vi "New Digital Edge Trigger.vi"(7 "Slope":T1, 8 "error in (no error)":errorcluster) -> (0 "error out":errorcluster, 3 "Digital Edge Trigger out":refnum<class "Digital Edge Trigger.lvclass">)   [LabVIEW 2015, in "Waveform Data Logger Engine.lvlib" / "Digital Edge Trigger.lvclass"]
uses:
  Digital Edge Trigger.lvclass
  Digital Slope Type.ctl
  Digital Edge Trigger.lvclass/Digital Edge Trigger.ctl
  Trigger/Trigger Type.ctl
  Trigger/Trigger.lvclass/Trigger.ctl
  Trigger/Write Trigger Type.vi
  Trigger/Trigger.lvclass
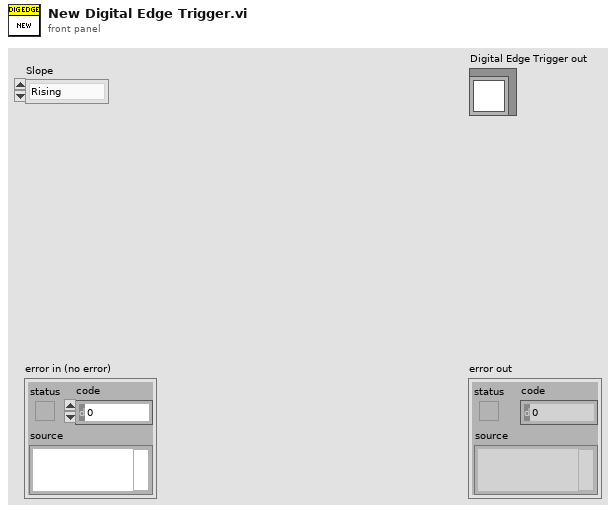
[diagram p1: front panel]
types:
  T1 = typedef "Waveform Data Logger Engine.lvlib/Digital Edge Trigger.lvclass/Digital Slope Type.ctl" = enum16{"Rising", "Falling"}
  T2 = typedef "Waveform Data Logger Engine.lvlib/Trigger.lvclass/Trigger Type.ctl" = enum16{"Default", "Digital Edge", "Analog Edge", "In Range", "Value Change", "Boolean Evaluation"}
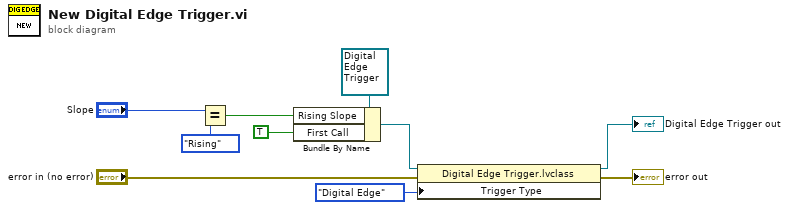
[diagram p0: block diagram]
diagram:
  n1 = Equal?(x="Slope", y=Digital_Slope_Type."Rising") -> (x = y?=w7:bool)
  n2 = Bundle By Name(cluster=refnum<class "Digital Edge Trigger.lvclass"> refnum ("Digital Edge Trigger in"), "Rising Slope"=w7, "First Call"=TRUE) -> (w2:refnum<class "Digital Edge Trigger.lvclass">)
  n3 = property class="Digital Edge Trigger.lvclass"(reference=w2, error in="error in (no error)", "Trigger Type"=Trigger_Type."Digital Edge") -> (reference out=→"Digital Edge Trigger out":refnum<class "Digital Edge Trigger.lvclass">, error out=→"error out":errorcluster)
